vi "Write PWM Delay.vi"(8 "error in (no error)":errorcluster, 10 "PWM Delay":dbl format="%.3g", 11 "Set Delay Msg in":refnum<class "Set Delay Msg.lvclass">) -> (0 "error out":errorcluster, 3 "Set Delay Msg out":refnum<class "Set Delay Msg.lvclass">)   [LabVIEW 2020, in "BNT_ULx.lvlib" / "Set Delay Msg.lvclass"]
uses:
  Set Delay Msg.lvclass
  Set Delay Msg.lvclass/Set Delay Msg.ctl
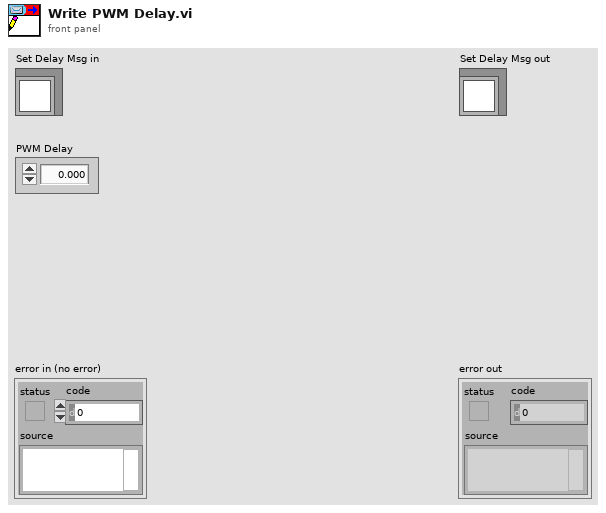
[diagram p1: front panel]
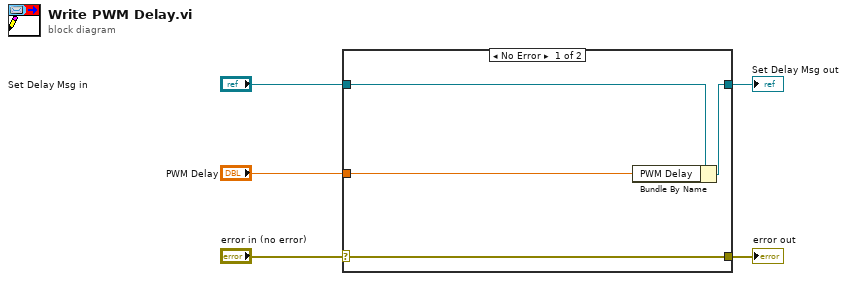
[diagram p0: block diagram]
diagram:
  n1 = case shown="No Error" "error in (no error)" {
    selector: "error in (no error)" -> [w9 w10]
    tunnel: [w9 w10] -> w4
    tunnel: [w7 w11] -> w2
    tunnel: "Set Delay Msg in" -> [w8 w11]
    tunnel: "PWM Delay" -> [w6 _]
    frame No Error {
      n2 = Bundle By Name(cluster=w8, "PWM Delay"=w6) -> (w7:refnum<class "Set Delay Msg.lvclass">)
    }
    frame Error {
    }
  }
  "error out" <- w4
  "Set Delay Msg out" <- w2
